vi "TCPReadI32.vi"(8 "error in (no error)":errorcluster, 9 "timeout ms (25000)":i32, 10 "command":string, 11 "connection ID":refnum<k5>) -> (0 "error out":errorcluster, 2 "I32 value":i32, 3 "connection ID out":refnum<k5>)   [LabVIEW 2013]
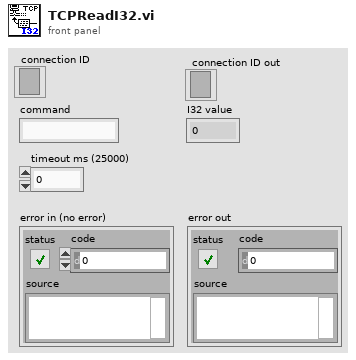
[diagram p1: front panel]
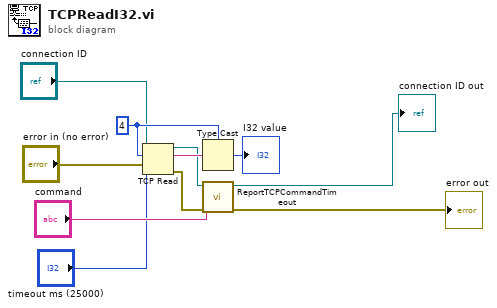
[diagram p0: block diagram]
diagram:
  w10 = 4 ("bytes to read")
  n1 = TCP Read(connection ID="connection ID", bytes to read=w10, error in (no error)="error in (no error)", 9:"timeout ms (25000)") -> (connection ID out=w8:refnum<k5>, data out=w11:string, error out=w9:errorcluster)  [unwired: 1 in]
  n2 = Type Cast(type=w10, x=w11) -> (*(type *) &x=→"I32 value":i32)
  n3 = call "ReportTCPCommandTimeout.vi"("error in (no error)"=w9, "command"="command", "connection ID"=w8) -> ("error out"=→"error out":errorcluster, "connection ID out"=→"connection ID out":refnum<k5>)  [unwired: 7 in]
